vi "getCodeElementsFromApplicationXMLFile.vi"(1 "Node":refnum<k20>) -> (0 "TextElements":T1)   [LabVIEW 2010]
uses:
  Program Files/National Instruments/LabVIEW 2010/resource/objmgr/DOMUserDefRef.rc
panel:
  out "XML":string
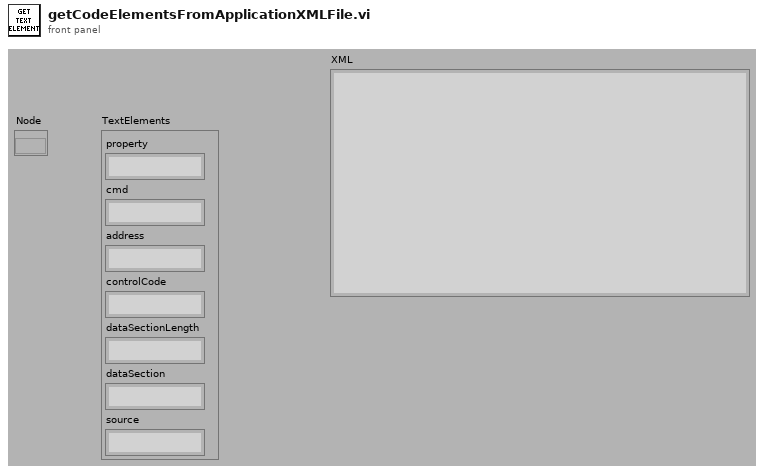
[diagram p1: front panel]
types:
  T1 = cluster{"property":string, "cmd":string, "address":string, "controlCode":string, "dataSectionLength":string, "dataSection":string, "source":string}
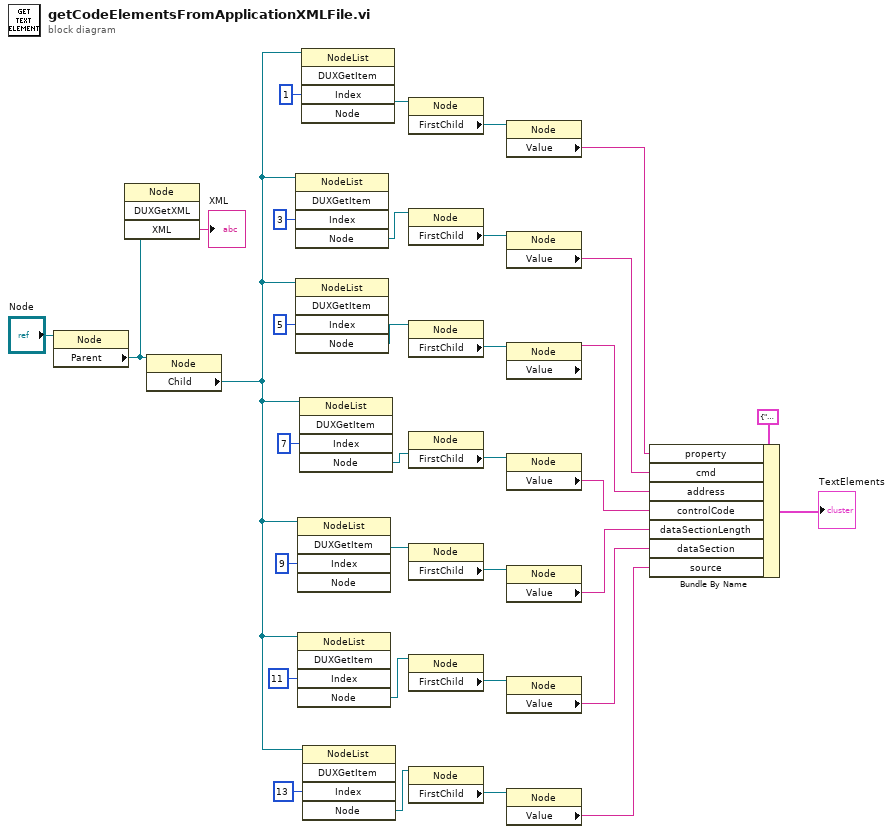
[diagram p0: block diagram]
diagram:
  n1 = property class="Node"(reference="Node") -> ("Parent"=w4:refnum<k20>)  [unwired: 1 in, 2 out]
  n2 = invoke class="Node" method="DUXGetXML"(reference=w4) -> ("XML"=→"XML":string)  [unwired: 3 in, 3 out]
  n3 = property class="Node"(reference=w4) -> ("Child"=w11:refnum<k20>)  [unwired: 1 in, 2 out]
  n4 = invoke class="NodeList" method="DUXGetItem"(reference=w11, "Index"=3) -> ("Node"=w13:refnum<k20>)  [unwired: 3 in, 4 out]
  n5 = invoke class="NodeList" method="DUXGetItem"(reference=w11, "Index"=5) -> ("Node"=w14:refnum<k20>)  [unwired: 3 in, 4 out]
  n6 = invoke class="NodeList" method="DUXGetItem"(reference=w11, "Index"=9) -> ("Node"=w18:refnum<k20>)  [unwired: 3 in, 4 out]
  n7 = invoke class="NodeList" method="DUXGetItem"(reference=w11, "Index"=11) -> ("Node"=w20:refnum<k20>)  [unwired: 3 in, 4 out]
  n8 = invoke class="NodeList" method="DUXGetItem"(reference=w11, "Index"=7) -> ("Node"=w16:refnum<k20>)  [unwired: 3 in, 4 out]
  n9 = invoke class="NodeList" method="DUXGetItem"(reference=w11, "Index"=1) -> ("Node"=w24:refnum<k20>)  [unwired: 3 in, 4 out]
  n10 = invoke class="NodeList" method="DUXGetItem"(reference=w11, "Index"=13) -> ("Node"=w22:refnum<k20>)  [unwired: 3 in, 4 out]
  n11 = property class="Node"(reference=w24) -> ("FirstChild"=w25:refnum<k20>)  [unwired: 1 in, 2 out]
  n12 = property class="Node"(reference=w13) -> ("FirstChild"=w12:refnum<k20>)  [unwired: 1 in, 2 out]
  n13 = property class="Node"(reference=w14) -> ("FirstChild"=w15:refnum<k20>)  [unwired: 1 in, 2 out]
  n14 = property class="Node"(reference=w16) -> ("FirstChild"=w17:refnum<k20>)  [unwired: 1 in, 2 out]
  n15 = property class="Node"(reference=w18) -> ("FirstChild"=w19:refnum<k20>)  [unwired: 1 in, 2 out]
  n16 = property class="Node"(reference=w20) -> ("FirstChild"=w21:refnum<k20>)  [unwired: 1 in, 2 out]
  n17 = property class="Node"(reference=w22) -> ("FirstChild"=w23:refnum<k20>)  [unwired: 1 in, 2 out]
  n18 = property class="Node"(reference=w25) -> ("Value"=w27:string)  [unwired: 1 in, 2 out]
  n19 = property class="Node"(reference=w12) -> ("Value"=w28:string)  [unwired: 1 in, 2 out]
  n20 = property class="Node"(reference=w15) -> ("Value"=w29:string)  [unwired: 1 in, 2 out]
  n21 = property class="Node"(reference=w17) -> ("Value"=w30:string)  [unwired: 1 in, 2 out]
  n22 = property class="Node"(reference=w19) -> ("Value"=w31:string)  [unwired: 1 in, 2 out]
  n23 = property class="Node"(reference=w21) -> ("Value"=w32:string)  [unwired: 1 in, 2 out]
  n24 = property class="Node"(reference=w23) -> ("Value"=w33:string)  [unwired: 1 in, 2 out]
  n25 = Bundle By Name(cluster=T1 {"property"="读通信地址", "cmd"="主站请求帧", "address"="############", "controlCode"="13", "dataSectionLength"="00", "dataSection"="无", "source"="主站"} ("TextElements"), "property"=w27, "cmd"=w28, "address"=w29, "controlCode"=w30, "dataSectionLength"=w31, "dataSection"=w32, "source"=w33) -> (→"TextElements":T1)
